vi "ZCAN_Receive.vi"(4 "error in (no error)":errorcluster caption="错误输入（无错误）", 7 "can_handle":u64) -> (0 "error out":errorcluster caption="错误输出", 1 "CANFD数据帧数组":T1(array[cluster]), 2 "CAN数据帧数组":T2(array[cluster]), 3 "Receive_Num":u32)   [LabVIEW 2018, in "zlgcan.lvlib"]
doc: "该函数用于接收CAN报文。"
uses:
  zlgcan.lvlib
  bin/ControlCANFD.dll
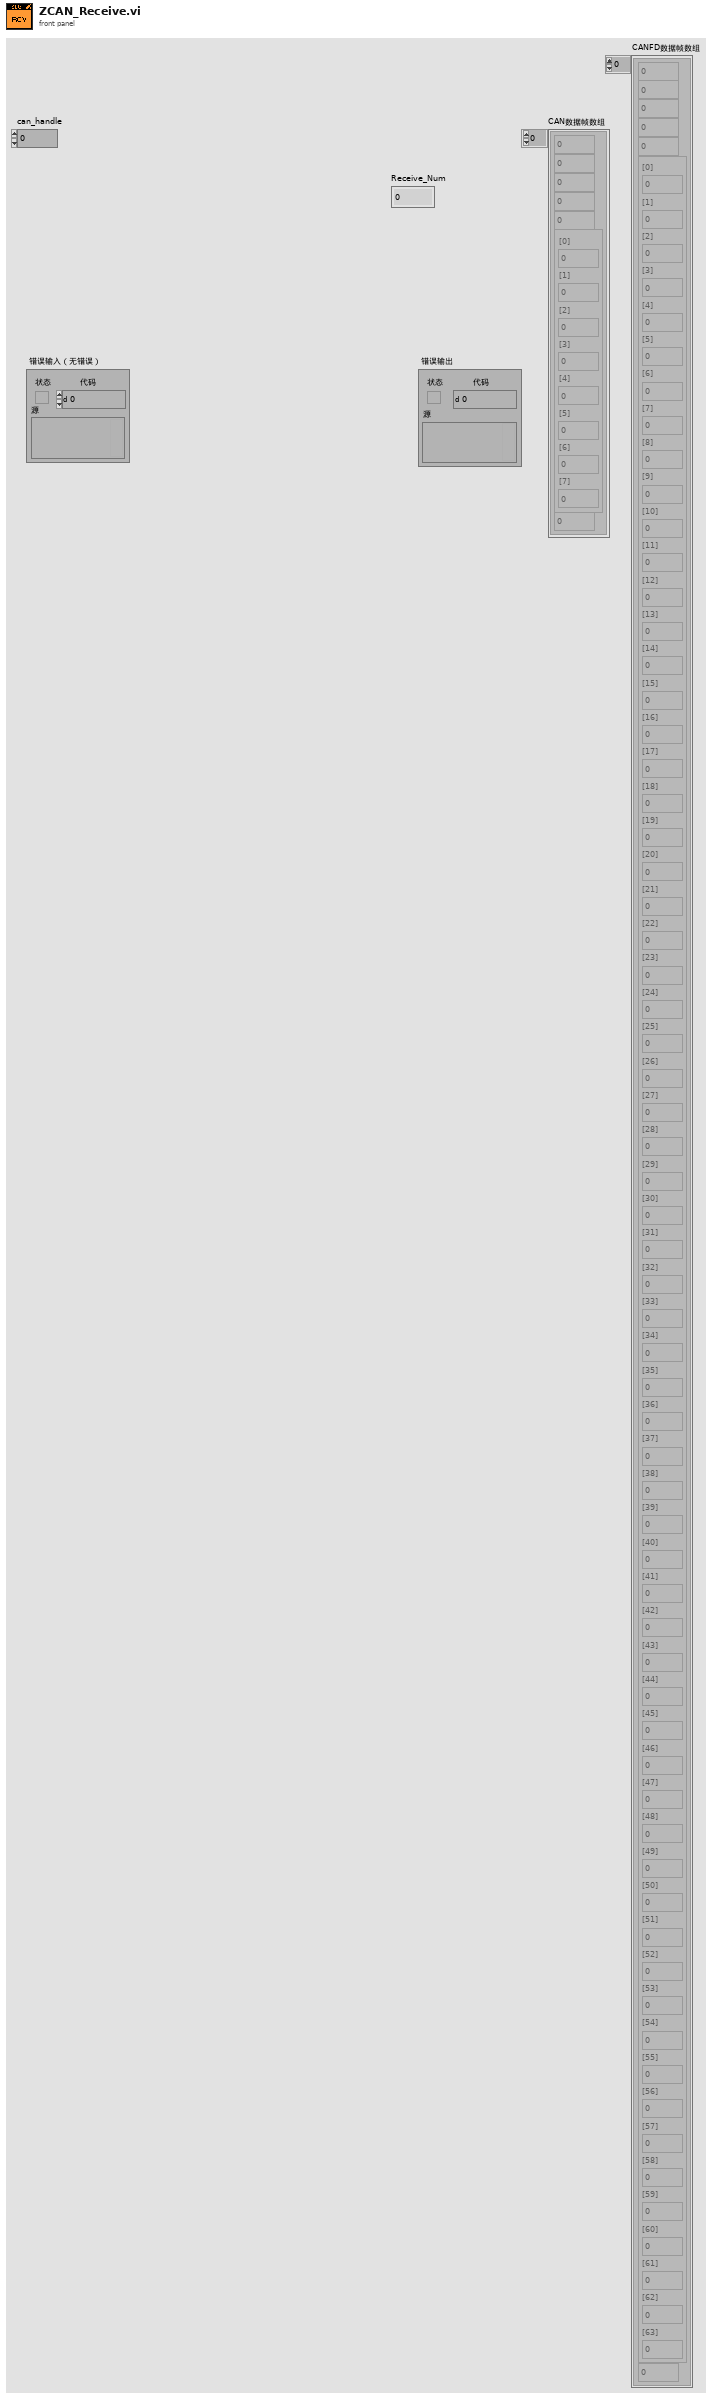
[diagram p1: front panel]
types:
  T1 = cluster{u32, u8, u8, u8, u8, cluster{"[0]":u8, "[1]":u8, "[2]":u8, "[3]":u8, "[4]":u8, "[5]":u8, "[6]":u8, "[7]":u8, "[8]":u8, "[9]":u8, "[10]":u8, "[11]":u8, "[12]":u8, "[13]":u8, "[14]":u8, "[15]":u8, "[16]":u8, "[17]":u8, "[18]":u8, "[19]":u8, "[20]":u8, "[21]":u8, "[22]":u8, "[23]":u8, "[24]":u8, "[25]":u8, "[26]":u8, "[27]":u8, "[28]":u8, "[29]":u8, "[30]":u8, "[31]":u8, "[32]":u8, "[33]":u8, "[34]":u8, "[35]":u8, "[36]":u8, "[37]":u8, "[38]":u8, "[39]":u8, "[40]":u8, "[41]":u8, "[42]":u8, "[43]":u8, "[44]":u8, "[45]":u8, "[46]":u8, "[47]":u8, "[48]":u8, "[49]":u8, "[50]":u8, "[51]":u8, "[52]":u8, "[53]":u8, "[54]":u8, "[55]":u8, "[56]":u8, "[57]":u8, "[58]":u8, "[59]":u8, "[60]":u8, "[61]":u8, "[62]":u8, "[63]":u8}, u64}[]
  T2 = cluster{u32, u8, u8, u8, u8, cluster{"[0]":u8, "[1]":u8, "[2]":u8, "[3]":u8, "[4]":u8, "[5]":u8, "[6]":u8, "[7]":u8}, u64}[]
  T3 = cluster{"[0]":u8, "[1]":u8, "[2]":u8, "[3]":u8, "[4]":u8, "[5]":u8, "[6]":u8, "[7]":u8, "[8]":u8, "[9]":u8, "[10]":u8, "[11]":u8, "[12]":u8, "[13]":u8, "[14]":u8, "[15]":u8, "[16]":u8, "[17]":u8, "[18]":u8, "[19]":u8, "[20]":u8, "[21]":u8, "[22]":u8, "[23]":u8, "[24]":u8, "[25]":u8, "[26]":u8, "[27]":u8, "[28]":u8, "[29]":u8, "[30]":u8, "[31]":u8, "[32]":u8, "[33]":u8, "[34]":u8, "[35]":u8, "[36]":u8, "[37]":u8, "[38]":u8, "[39]":u8, "[40]":u8, "[41]":u8, "[42]":u8, "[43]":u8, "[44]":u8, "[45]":u8, "[46]":u8, "[47]":u8, "[48]":u8, "[49]":u8, "[50]":u8, "[51]":u8, "[52]":u8, "[53]":u8, "[54]":u8, "[55]":u8, "[56]":u8, "[57]":u8, "[58]":u8, "[59]":u8, "[60]":u8, "[61]":u8, "[62]":u8, "[63]":u8}
  T4 = cluster{u32, u8, u8, u8, u8, cluster{"[0]":u8, "[1]":u8, "[2]":u8, "[3]":u8, "[4]":u8, "[5]":u8, "[6]":u8, "[7]":u8, "[8]":u8, "[9]":u8, "[10]":u8, "[11]":u8, "[12]":u8, "[13]":u8, "[14]":u8, "[15]":u8, "[16]":u8, "[17]":u8, "[18]":u8, "[19]":u8, "[20]":u8, "[21]":u8, "[22]":u8, "[23]":u8, "[24]":u8, "[25]":u8, "[26]":u8, "[27]":u8, "[28]":u8, "[29]":u8, "[30]":u8, "[31]":u8, "[32]":u8, "[33]":u8, "[34]":u8, "[35]":u8, "[36]":u8, "[37]":u8, "[38]":u8, "[39]":u8, "[40]":u8, "[41]":u8, "[42]":u8, "[43]":u8, "[44]":u8, "[45]":u8, "[46]":u8, "[47]":u8, "[48]":u8, "[49]":u8, "[50]":u8, "[51]":u8, "[52]":u8, "[53]":u8, "[54]":u8, "[55]":u8, "[56]":u8, "[57]":u8, "[58]":u8, "[59]":u8, "[60]":u8, "[61]":u8, "[62]":u8, "[63]":u8}, u64}
  T5 = cluster{"[0]":u8, "[1]":u8, "[2]":u8, "[3]":u8, "[4]":u8, "[5]":u8, "[6]":u8, "[7]":u8}
  T6 = cluster{u32, u8, u8, u8, u8, cluster{"[0]":u8, "[1]":u8, "[2]":u8, "[3]":u8, "[4]":u8, "[5]":u8, "[6]":u8, "[7]":u8}, u64}
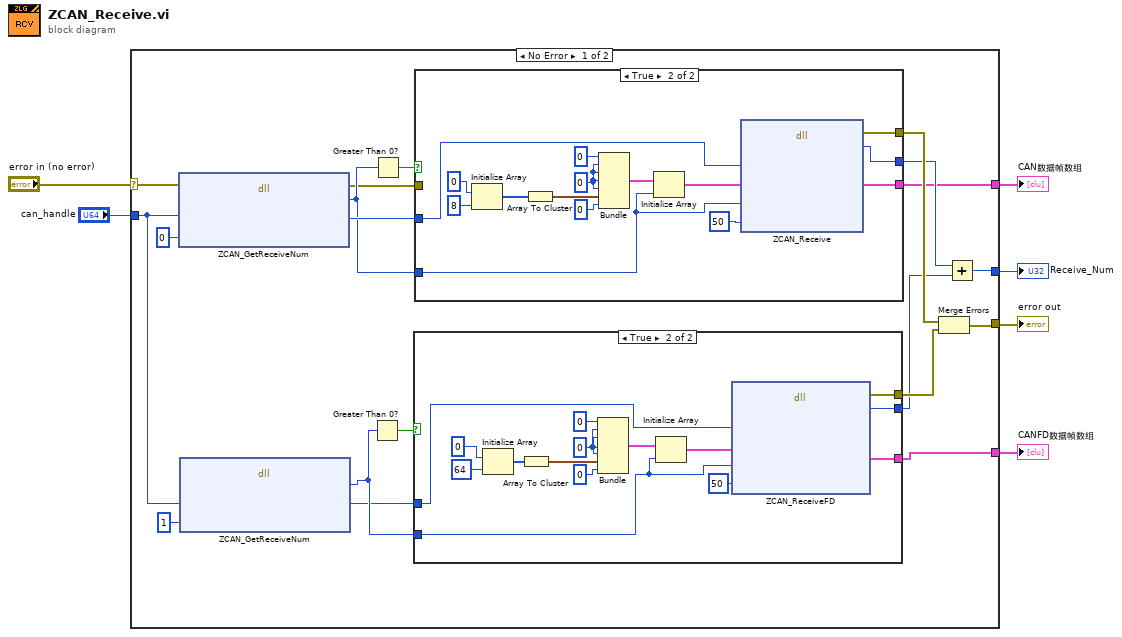
[diagram p0: block diagram]
diagram:
  n1 = case shown="No Error" "error in (no error)" {
    selector: "error in (no error)" -> [w25 w56]
    tunnel: [w14 w56] -> w5
    tunnel: "can_handle" -> [w19 _]
    tunnel: [w11 _] -> w3
    tunnel: [w10 _] -> w2
    tunnel: [w9 _] -> w1
    frame No Error {
      n2 = dll-call lib="C:/Users/ttc52/Desktop/DHC FD LV2018/LABIVIEW CANFD Tool_V1.2.4_20220724/bin/ControlCANFD.dll" fn="ZCAN_GetReceiveNum"(error in=w25, "通道句柄"=w19, "协议"=u8 0) -> (error out=w7:errorcluster, "缓冲区帧数"=w22:u32, "通道句柄"=w23:u64)  [unwired: 3 in, 1 out]
      n3 = dll-call lib="C:/Users/ttc52/Desktop/DHC FD LV2018/LABIVIEW CANFD Tool_V1.2.4_20220724/bin/ControlCANFD.dll" fn="ZCAN_GetReceiveNum"("通道句柄"=w19, "协议"=u8 1) -> ("缓冲区帧数"=w17:u32, "通道句柄"=w8:u64)  [unwired: 4 in, 2 out]
      n4 = Greater Than 0?(x=w17) -> (x > 0?=w18:bool)
      n5 = Greater Than 0?(x=w22) -> (x > 0?=w24:bool)
      n6 = case shown="True" w18 {
        tunnel: w17 -> [_ w29]
        tunnel: [_ w39] -> w9
        tunnel: [_ w38] -> w15
        tunnel: [_ w26] -> w13
        tunnel: w8 -> [_ w27]
        frame False {
        }
        frame True {
          w33 = u8 0
          n7 = Initialize Array(u8 0 ("元素"), u32 64 ("维数大小")) -> (w35:u8[])
          n8 = Array To Cluster(array=w35) -> (cluster=w36:T3)
          n9 = Bundle(u32 0, w33, w33, w33, w33, w36, u64 0) -> (w37:T4)  [unwired: 1 in]
          n10 = Initialize Array(w37, w29) -> (w28:T1)
          n11 = dll-call lib="C:/Users/ttc52/Desktop/DHC FD LV2018/LABIVIEW CANFD Tool_V1.2.4_20220724/bin/ControlCANFD.dll" fn="ZCAN_ReceiveFD"("通道句柄"=w27, "数据帧数组"=w28, "数据帧数"=w29, "超时时间"=50) -> (error out=w38:errorcluster, "已接收帧数"=w26:u32, "数据帧数组"=w39:T1)  [unwired: 6 in, 1 out]
        }
      }
      n12 = case shown="True" w24 {
        tunnel: w23 -> [_ w45]
        tunnel: w22 -> [_ w44]
        tunnel: [_ w43] -> w10
        tunnel: [_ w42] -> w16
        tunnel: [_ w41] -> w12
        tunnel: w7 -> [_ _]
        frame False {
        }
        frame True {
          w51 = u8 0
          n13 = Initialize Array(u8 0 ("元素"), u32 8 ("维数大小")) -> (w53:u8[])
          n14 = Array To Cluster(array=w53) -> (cluster=w54:T5)
          n15 = Bundle(u32 0, w51, w51, w51, w51, w54, u64 0) -> (w55:T6)  [unwired: 1 in]
          n16 = Initialize Array(w55, w44) -> (w46:T2)
          n17 = dll-call lib="C:/Users/ttc52/Desktop/DHC FD LV2018/LABIVIEW CANFD Tool_V1.2.4_20220724/bin/ControlCANFD.dll" fn="ZCAN_Receive"("通道句柄"=w45, "数据帧数组"=w46, "数据帧数"=w44, "超时时间"=50) -> (error out=w42:errorcluster, "已接收帧数"=w41:u32, "数据帧数组"=w43:T2)  [unwired: 6 in, 1 out]
        }
      }
      n18 = Merge Errors(w16, w15) -> (w14:errorcluster)
      n19 = Add(x=w12, y=w13) -> (x+y=w11:u32)
    }
    frame Error {
    }
  }
  "error out" <- w5
  "Receive_Num" <- w3
  "CAN数据帧数组" <- w2
  "CANFD数据帧数组" <- w1
